vi "simple_PID.vi"(4 "lower limit":dbl format="%0.2f", 6 "upper limit":dbl format="%0.2f", 7 "process variable":dbl format="%0.2f", 8 "D":dbl=0.05 format="%0.2f", 9 "I":dbl=0.1 format="%0.2f", 10 "P":dbl=1.0 format="%0.2f", 11 "set point":dbl format="%0.2f") -> (3 "output value":dbl caption="output value 2" format="%0.2f")   [LabVIEW 2010]
doc: "This is a simple PID which can be used to control a system. The idea of a PID is to control a system by comparing the set point (the system value you want) to the process variable (the current system value), and adjusting the output value (what you output to the system in an attempt to get the process variable to approach the set point.\n\nThe set point is the value you desire the system to achieve.\n\nThe process variable is the current value of your system, and is usually acquired by an analog input channel of your DAQ device.\n\nP is the Proportional component. This is the amount by which the error gets multiplied. The error is the set point minus the process variable.\n\nI is the Integral component. This is how much the PID output will depend on what has happened in the past.\n\nD is the derivative component. This is how much the PID output will depend on speculation of what will happen in the future.\n\nThe output value is the PID output which is usually generated at an analog output channel of your DAQ device in an attempt to get the process variable equal to the set point.\n\nThe upper limit is the maximum value the PID can output to the system.\n\nThe lower limit is the minimum value the PID can output to the system."
panel:
  # "Note: This function is not designed for control\nloop rates > 1kHz.  The dt calcuation has a\nresolution of 1 ms, therefore loop rates > 1kHz\nwill result in incorrect output for derivative and\nintegral action."
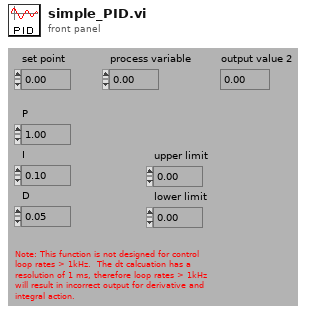
[diagram p1: front panel]
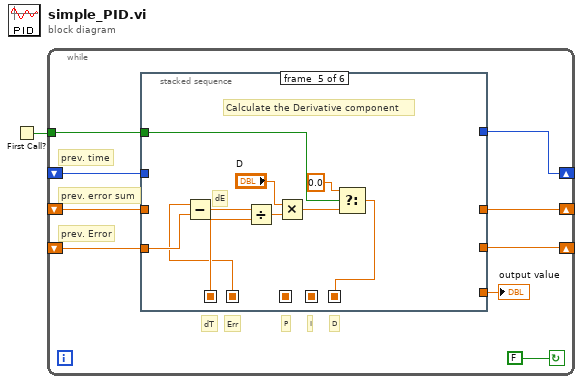
[diagram p0: block diagram]
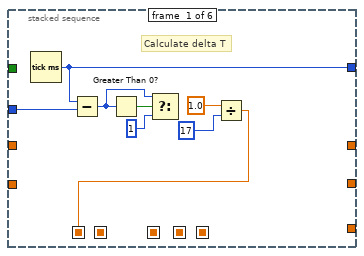
[diagram p2: hidden frame]
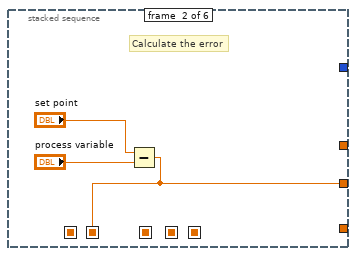
[diagram p3: hidden frame]
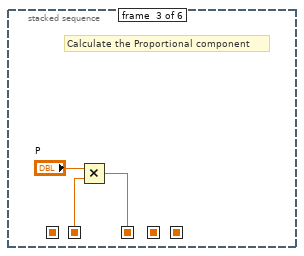
[diagram p4: hidden frame]
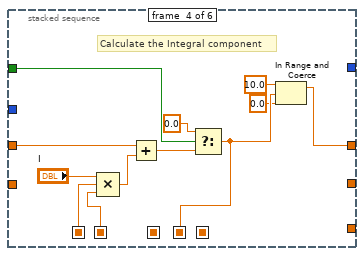
[diagram p5: hidden frame]
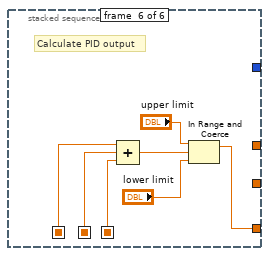
[diagram p6: hidden frame]
diagram:
  n1 = First Call?() -> (First Call?: T/F=w1:bool)
  n2 = while {
    shift-left: _ -> [w5]
    shift-right: [w6] -> _
    shift-left: _ -> [w8]
    shift-right: [w7] -> _
    shift-left: _ -> [w9]
    shift-right: [w10] -> _
    tunnel: w1 -> [w2]
    stop <- FALSE continue-if-true
    # "I"
    # "dT"
    # "Err"
    # "D"
    # "P"
    # "prev. error sum"
    # "prev. time"
    # "prev. Error"
    n3 = stacked-sequence {
      seq-local: [w12 _ _ _ _ _] -> [_ _ _ w32 w41 _]
      seq-local: [_ w19 _ _ _ _] -> [_ _ w23 w31 w40 _]
      seq-local: [_ _ w22 _ _ _] -> [_ _ _ _ _ w52]
      seq-local: [_ _ _ _ w39 _] -> [_ _ _ _ _ w50]
      seq-local: [_ _ _ w28 _ _] -> [_ _ _ _ _ w51]
      tunnel: [w13 _ _ _ _ _] -> w10
      tunnel: w9 -> [w14 _ _ _ _ _]
      tunnel: w8 -> [_ _ _ w33 _ _]
      tunnel: [_ _ _ w27 _ _] -> w7
      tunnel: [_ w19 _ _ _ _] -> w6
      tunnel: w5 -> [_ _ _ _ w42 _]
      tunnel: [_ _ _ _ _ w49] -> w4
      tunnel: w2 -> [_ _ _ w30 w38 _]
      frame #0 {
        # "Calculate delta T"
        n4 = Tick Count (ms)() -> (millisecond timer value=w13:u32)
        n5 = Subtract(x=w13, y=w14) -> (x-y=w17:u32)
        n6 = Greater Than 0?(x=w17) -> (x > 0?=w18:bool)
        n7 = Select(t=w17, s=w18, f=u32 1) -> ()  [unwired: 1 out]
        n8 = Divide(x=1.0, y=17) -> (x/y=w12:dbl)
      }
      frame #1 {
        # "Calculate the error"
        n9 = Subtract(x="set point", y="process variable") -> (x-y=w19:dbl)
      }
      frame #2 {
        # "Calculate the Proportional component"
        n10 = Multiply(x="P", y=w23) -> (x*y=w22:dbl)
      }
      frame #3 {
        # "Calculate the Integral component"
        n11 = Compound Arithmetic op=MULTIPLY("I", w32, w31) -> (w36:dbl)
        n12 = Add(x=w33, y=w36) -> (x+y=w34:dbl)
        n13 = Select(t=0.0, s=w30, f=w34) -> (s? t:f=w28:dbl)
        n14 = In Range and Coerce(upper limit=10.0 ("Obergrenze"), x=w28, lower limit=0.0 ("Untergrenze")) -> (coerced(x)=w27:dbl)  [unwired: 1 out]
      }
      frame #4 {
        # "dE"
        # "Calculate the Derivative component"
        n15 = Subtract(x=w40, y=w42) -> (x-y=w43:dbl)
        n16 = Divide(x=w43, y=w41) -> (x/y=w44:dbl)
        n17 = Multiply(x="D", y=w44) -> (x*y=w46:dbl)
        n18 = Select(t=0.0, s=w38, f=w46) -> (s? t:f=w39:dbl)
      }
      frame #5 {
        # "Calculate PID output"
        n19 = Compound Arithmetic op=ADD(w52, w51, w50) -> (w53:dbl)
        n20 = In Range and Coerce(upper limit="upper limit", x=w53, lower limit="lower limit") -> (coerced(x)=w49:dbl)  [unwired: 1 out]
      }
    }
    "output value" <- w4
  }
